vi "SetShutterStatus.vi"(8 "error in (no error)":errorcluster, 9 "Value":bool, 10 "Label":string, 11 "Laser_Oxxius in":refnum<class "Laser_Oxxius.lvclass">) -> (0 "error out":errorcluster, 3 "Laser_Oxxius out":refnum<class "Laser_Oxxius.lvclass">)   [LabVIEW 2020, in "Laser_Oxxius.lvlib" / "Laser_Oxxius.lvclass"]
uses:
  Laser_Oxxius.lvclass
  Laser_Oxxius.lvclass/Laser_Oxxius.ctl
  D:/Daguan/Development/MMicroscopyAF/Model/Real Hardware/Laser_Oxxius/Laser_Oxxius/Dependency/Oxxius_Boxx.dll
  Dependency/Oxxius_Boxx.dll
  HAL Layer/Component/Laser/Laser/Laser.lvclass
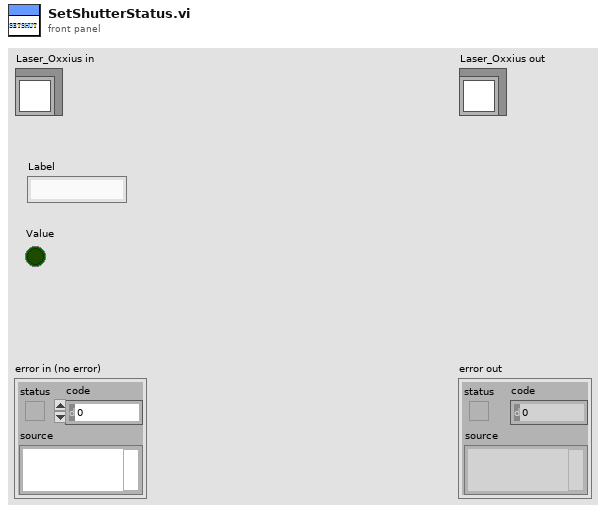
[diagram p1: front panel]
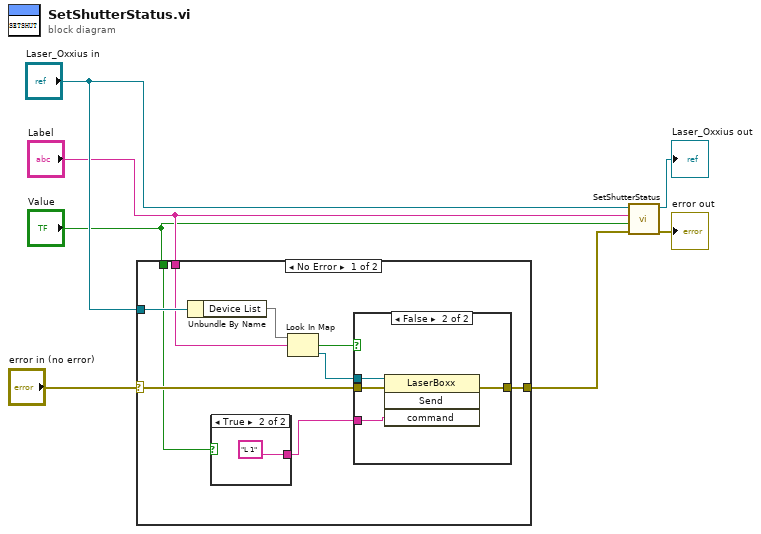
[diagram p0: block diagram]
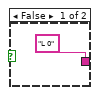
[diagram p2: hidden frame]
diagram:
  n1 = case shown="No Error" "error in (no error)" {
    selector: "error in (no error)" -> [w16 w24]
    tunnel: "Laser_Oxxius in" -> [w15 _]
    tunnel: [w11 w24] -> w4
    tunnel: "Value" -> [w9 _]
    tunnel: "Label" -> [w13 _]
    frame No Error {
      n2 = Unbundle By Name(w15) -> ("Device List"=w14:map{string, refnum<k24>})
      n3 = case shown="True" w9 {
        tunnel: ["L 0" ("command") "L 1" ("command")] -> w8
        frame False {
        }
        frame True {
        }
      }
      n4 = Look In Map(map=w14, key=w13) -> (key not found?=w10:bool, value=w12:refnum<k24>)  [unwired: 1 in]
      n5 = case shown="False" w10 {
        tunnel: w16 -> [w19 w23]
        tunnel: w12 -> [_ w22]
        tunnel: [w19 w21] -> w11
        tunnel: w8 -> [_ w20]
        frame True {
        }
        frame False {
          n6 = invoke class="LaserBoxx" method="Send"(reference=w22, error in=w23, "command"=w20) -> (error out=w21:errorcluster)  [unwired: 1 in, 3 out]
        }
      }
    }
    frame Error {
    }
  }
  n7 = call-parent "SetShutterStatus.vi"("error in (no error)"=w4, "Value"="Value", "Label"="Label", "Laser in"="Laser_Oxxius in") -> ("error out"=→"error out":errorcluster, "Laser out"=→"Laser_Oxxius out":refnum<class "Laser_Oxxius.lvclass">)  [unwired: 6 in]
